vi "GetSignalByName.vi"(10 "Signal Name":string, 11 "Signal Array Input":T1[](array[typedef])) -> (3 "Retreived Signal":T1)   [LabVIEW 2016]
uses:
  Ctrl_Signal.ctl
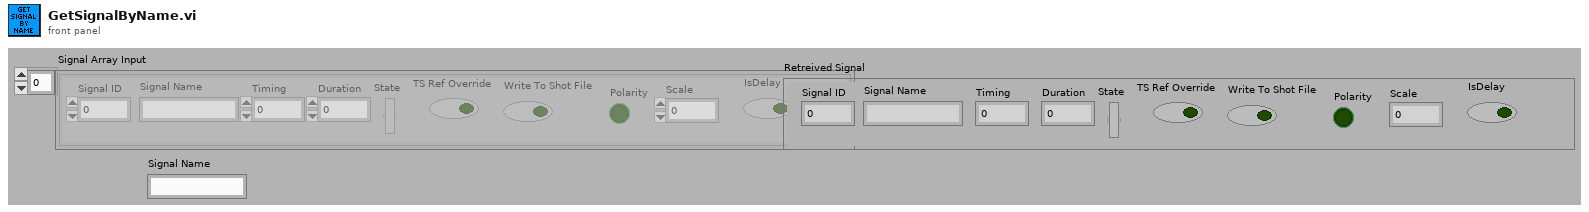
[diagram p1: front panel]
types:
  T1 = typedef "Ctrl_Signal.ctl" = cluster{"Signal Name":string, "Timing":dbl, "Duration":dbl, "State":bool, "TS Ref Override":bool, "Write To Shot File":bool, "Polarity":bool, "Signal ID":dbl, "Scale":dbl, "IsDelay":bool}
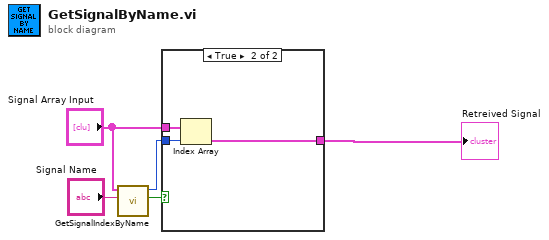
[diagram p0: block diagram]
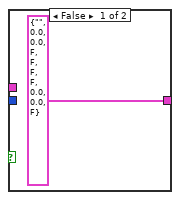
[diagram p2: hidden frame]
diagram:
  n1 = call "GetSignalIndexByName.vi"("Signal Name"="Signal Name", "Signal Array In"="Signal Array Input") -> ("Signal Found"=w4:bool, "Index Out"=w2:u32)  [unwired: 8 in]
  n2 = case shown="True" w4 {
    tunnel: "Signal Array Input" -> [_ w9]
    tunnel: w2 -> [_ w8]
    tunnel: [T1 {"Signal Name"="", "Timing"=0.0, "Duration"=0.0, "State"=FALSE, "TS Ref Override"=FALSE, "Write To Shot File"=FALSE, "Polarity"=FALSE, "Signal ID"=0.0, "Scale"=0.0, "IsDelay"=FALSE} ("Ctrl_Signal") w7] -> w1
    frame False {
    }
    frame True {
      n3 = Index Array(array=w9, index=w8) -> (element=w7:T1)
    }
  }
  "Retreived Signal" <- w1
